vi "Connect to DB Example.vi"() -> ()   [LabVIEW 2018, in "Database.lvlib"]
uses:
  Database.lvlib
  DatabaseBaseClass/DatabaseBaseClass.lvclass
  AcPwr/AcPwrPlugins/ChromaPowerSupplyModelClass/TypeDefs/ChromaPS_ICDAS2Model.ctl
  AcPwr/AcPwrPlugins/ChromaPowerSupplyModelClass/TypeDefs/ChromaPS_Model2ICDAS.ctl
  AcPwr/AcPwrPlugins/ChromaPowerSupplyModelClass/ChromaPowerSupplyModel.lvclass
panel:
  in  "DatabaseBaseClass in":refnum<class "DatabaseBaseClass.lvclass">
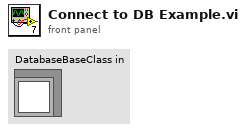
[diagram p1: front panel]
types:
  T1 = typedef "AcPwrPlugins.lvlib/ChromaPowerSupplyModel.lvclass/ChromaPS_Model2ICDAS.ctl" = cluster{"data_id":i32, "voltage":dbl, "current":dbl, "power":dbl, "meas_timestamp":timestamp, "write_timestamp":timestamp, "read_by_icdas":bool, "read_timestamp":timestamp}
  T2 = typedef "AcPwrPlugins.lvlib/ChromaPowerSupplyModel.lvclass/ChromaPS_ICDAS2Model.ctl" = cluster{"data_id":i32, "data":string, "write_timestamp":timestamp, "read_by_model":bool, "read_timestamp":timestamp}
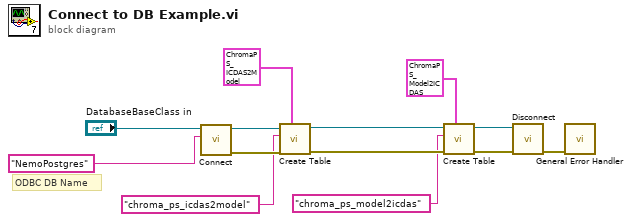
[diagram p0: block diagram]
diagram:
  # "ODBC DB Name"
  n1 = call-dynamic "Connect.vi"("Data Source"="NemoPostgres" ("connection information"), "DatabaseBaseClass in"="DatabaseBaseClass in") -> ("error out"=w11:errorcluster, "DatabaseBaseClass out"=w13:refnum<class "DatabaseBaseClass.lvclass">)  [unwired: 8 in]
  n2 = call-dynamic "Create Table.vi"("Cluster In"=T2 {"data_id"=0, "data"="", "write_timestamp"=timestamp(0 s since 1904-01-01), "read_by_model"=FALSE, "read_timestamp"=timestamp(0 s since 1904-01-01)} ("ACDCDifferenceData"), "error in (no error)"=w11, "Table Name"="chroma_ps_icdas2model", "DatabaseBaseClass In"=w13) -> ("error out"=w8:errorcluster, "DatabaseBaseClass out"=w7:refnum<class "DatabaseBaseClass.lvclass">)  [unwired: 4 in, 2 out]
  n3 = call-dynamic "Create Table.vi"("Cluster In"=T1 {"data_id"=0, "voltage"=0.0, "current"=0.0, "power"=0.0, "meas_timestamp"=timestamp(0 s since 1904-01-01), "write_timestamp"=timestamp(0 s since 1904-01-01), "read_by_icdas"=FALSE, "read_timestamp"=timestamp(0 s since 1904-01-01)} ("Calibration Table"), "error in (no error)"=w8, "Table Name"="chroma_ps_model2icdas", "DatabaseBaseClass In"=w7) -> ("error out"=w4:errorcluster, "DatabaseBaseClass out"=w3:refnum<class "DatabaseBaseClass.lvclass">)  [unwired: 4 in, 2 out]
  n4 = call-dynamic "Disconnect.vi"("error in (no error)"=w4, "DatabaseBaseClass in"=w3) -> ("error out"=w2:errorcluster)  [unwired: 8 in, 1 out]
  n5 = call <vilib>:"General Error Handler.vi"("error in (no error)"=w2) -> ()  [unwired: 10 in, 5 out]
